vi "Configure System.vi"(0 "VISA resource name":refnum<visa-resource-name>, 1 "Autozero Enabled? (T: On)":bool=TRUE, 2 "Beeper Enabled? (T: On)":bool=TRUE, 5 "error in (no error)":errorcluster) -> (14 "VISA resource name out":refnum<visa-resource-name>, 19 "error out":errorcluster)   [LabVIEW 2018, in "Keithley 2000.lvlib"]
doc: "This VI configures various system settings on the instrument. This includes enabling or disabling autozeroing and the beeper.\n\nNote:\nThis VI aborts the trigger system."
uses:
  <instrlib>/Keithley 2000/Keithley 2000.lvlib
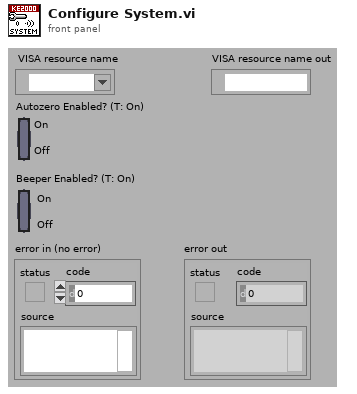
[diagram p1: front panel]
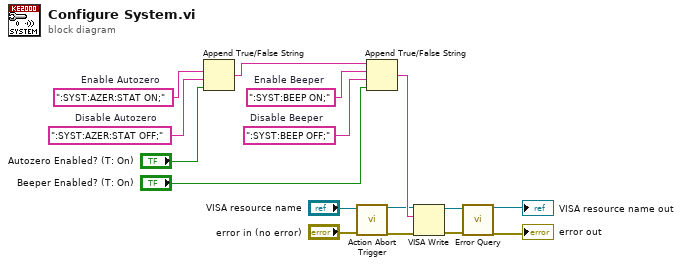
[diagram p0: block diagram]
diagram:
  w13 = ":SYST:BEEP OFF;"  # Disable Beeper
  w14 = ":SYST:BEEP ON;"  # Enable Beeper
  w15 = ":SYST:AZER:STAT OFF;"  # Disable Autozero
  w16 = ":SYST:AZER:STAT ON;"  # Enable Autozero
  n1 = Append True/False String(1:"Autozero Enabled? (T: On)", 2:w15, 3:w16) -> (0:w12:string)  [unwired: 1 in]
  n2 = call <instrlib>:"Action Abort Trigger.vi"("VISA resource name"="VISA resource name", "error in (no error)"="error in (no error)") -> ("VISA resource name out"=w5:refnum<visa-resource-name>, "error out"=w6:errorcluster)  [unwired: 16 in]
  n3 = Append True/False String(1:"Beeper Enabled? (T: On)", 2:w13, 3:w14, 4:w12) -> (0:w11:string)
  n4 = VISA Write(VISA resource name=w5, write buffer=w11, error in (no error)=w6) -> (VISA resource name out=w4:refnum<visa-resource-name>, error out=w1:errorcluster)  [unwired: 1 out]
  n5 = call <instrlib>:"Error Query.vi"("VISA resource name"=w4, "error in (no error)"=w1) -> ("VISA resource name out"=→"VISA resource name out":refnum<visa-resource-name>, "error out"=→"error out":errorcluster)  [unwired: 14 in, 2 out]
